vi "Terminate.vi"(8 "error in (no error)":errorcluster, 10 "Message in":refnum<class "TerminateMessage.lvclass">, 11 "Waveform in":refnum<class "Waveform.lvclass">) -> (0 "error out":errorcluster, 3 "Waveform out":refnum<class "Waveform.lvclass">)   [LabVIEW 2012, in "Waveform.lvclass"]
doc: "This member function is called when the statemachine in the run.vi receives an 'terminate' command. It closes the RabbitMQ connection. \n\nOverride this member function in your derived class to release all previously acquired resources (but don't forget to call the parent method). If your component has subcomponents, they count as resources, and you have to release them by calling their own terminate functions."
uses:
  Waveform.lvclass
  <vilib>/Distrio/Murmex/TerminateMessage/TerminateMessage.lvclass
  Waveform.lvclass/Waveform.ctl
  <vilib>/Distrio/Murmex/Murmex/Murmex.lvclass
panel:
  # "This method is called when the TERMINATE\ntrigger is sent. \n\nOverride this method when your component needs to\nrespond to this trigger. \n\nCall parent for proper implementation"
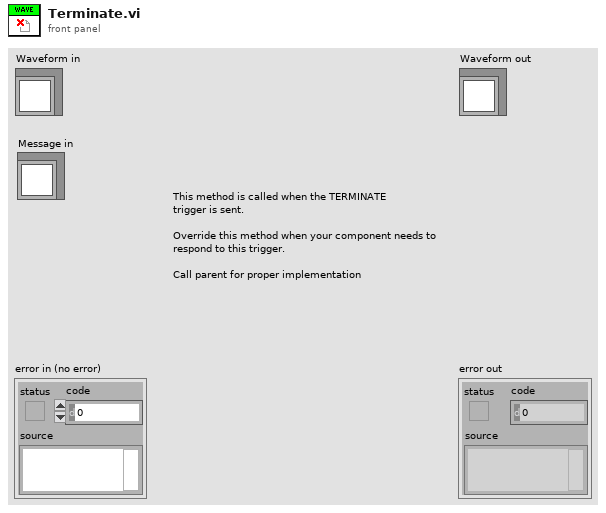
[diagram p1: front panel]
types:
  T1 = enum8{"Enabled", "Disabled", "Disabled and Grayed Out"}
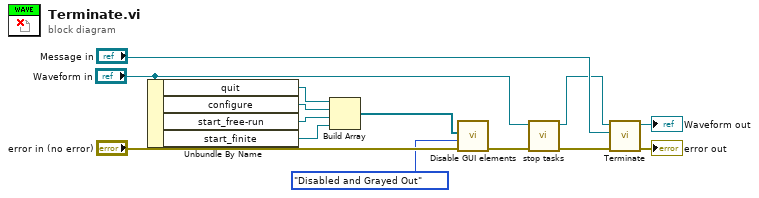
[diagram p0: block diagram]
diagram:
  n1 = Unbundle By Name("Waveform in") -> ("quit"=w9:refnum<vi>, "configure"=w8:refnum<vi>, "start_free-run"=w7:refnum<vi>, "start_finite"=w6:refnum<vi>)
  n2 = Build Array(w9, w8, w7, w6) -> (w5:refnum<vi>[])
  n3 = call <vilib>:"Disable GUI elements.vi"("error in (no error)"="error in (no error)", "enabled state"=T1."Disabled and Grayed Out", "control refs"=w5) -> ("error out"=w4:errorcluster)  [unwired: 8 in]
  n4 = call-dynamic "stop tasks.vi"("error in (no error)"=w4, "Waveform in"="Waveform in") -> ("error out"=w3:errorcluster, "Waveform out"=w1:refnum<class "Waveform.lvclass">)  [unwired: 8 in]
  n5 = call-parent "Terminate.vi"("error in (no error)"=w3, "Message in"="Message in", "Murmex in"=w1) -> ("error out"=→"error out":errorcluster, "Murmex out"=→"Waveform out":refnum<class "Waveform.lvclass">)  [unwired: 7 in]
